vi "File_header_diag_Hall.vi"(0 "Byte Stream File in":refnum<file>, 2 "SteppingMode":dbl, 3 "OFFSET":dbl, 4 "Sample area":dbl, 5 "Gain":dbl, 6 "Averaging":dbl, 10 "DwellTime":dbl, 13 "Reoffset":dbl, 14 "Stabilization time":dbl, 15 "Window":dbl) -> ()   [LabVIEW 2015]
uses:
  <vilib>/Utility/file.llb/Write Delimited Spreadsheet (string).vi
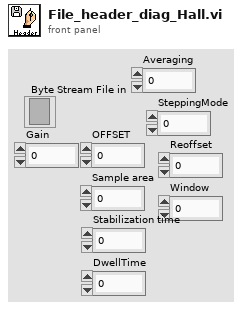
[diagram p1: front panel]
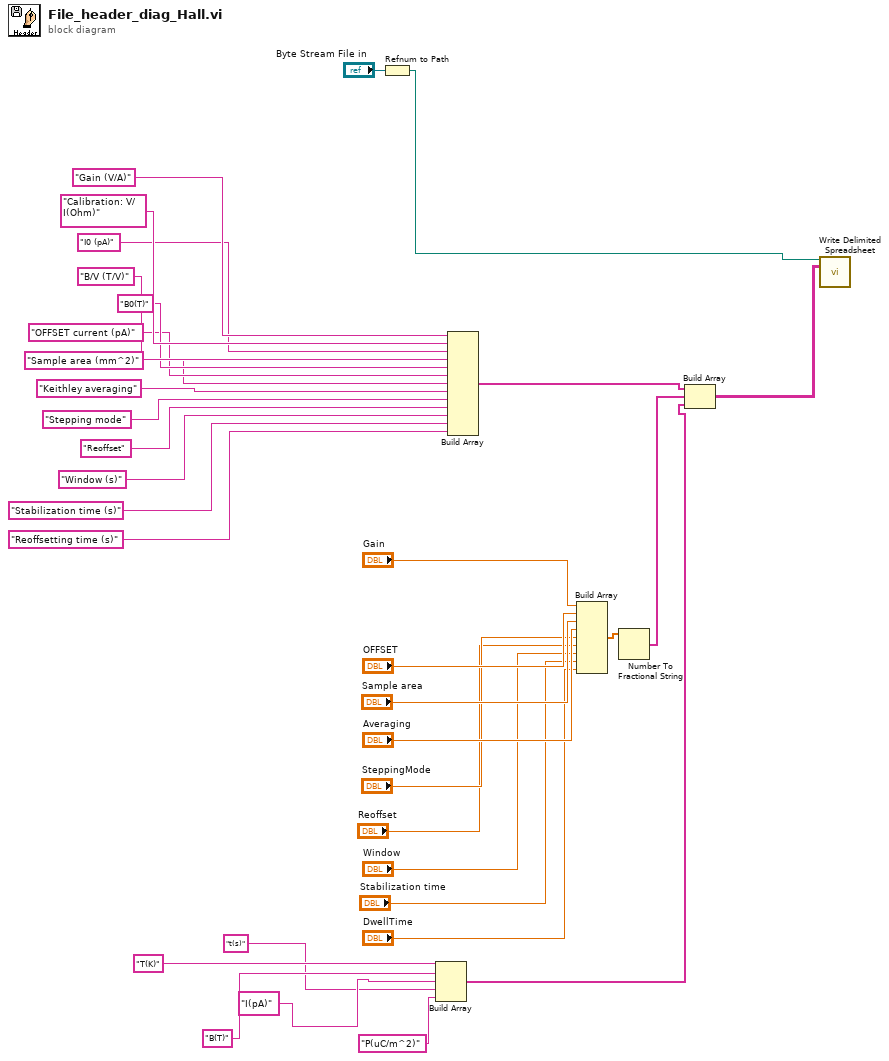
[diagram p0: block diagram]
diagram:
  n1 = Refnum to Path(1:"Byte Stream File in") -> (0:w33:path)
  n2 = Build Array("T(K)" ("element"), "B(T)", "I(pA)", "t(s)", "P(uC/m^2)" ("element")) -> (w18:string[])
  n3 = Build Array("Gain (V/A)" ("element"), "Calibration: V/I(Ohm)", "I0 (pA)", "B/V (T/V)" ("element"), "B0(T)", "OFFSET current (pA)" ("element"), "Sample area (mm^2)" ("element"), "Keithley averaging" ("element"), "Stepping mode" ("element"), "Reoffset" ("element"), "Window (s)" ("element"), "Stabilization time (s)" ("element"), "Reoffsetting time (s)" ("element")) -> (w20:string[])
  n4 = Build Array("Gain", "OFFSET", "Sample area", "Averaging", "SteppingMode", "Reoffset", "Window", "Stabilization time", "DwellTime") -> (w21:dbl[])
  n5 = Number To Fractional String(number=w21) -> (F-format string=w19:string[])  [unwired: 3 in]
  n6 = Build Array(w20, w19, w18) -> (w17:string[][])
  n7 = call-poly <vilib>:"Write Delimited Spreadsheet.vi"("file path (dialog if empty)"=w33, "2D data"=w17) -> ()  [unwired: 12 in, 2 out]
